vi "Memory.Pointer.Allocate.vi"(7 "allocation limit (2^31: 2GiB)":u64=2147483647 format="%08x bytes", 8 "error in (no error)":errorcluster, 10 "size":u64 format="%d bytes", 11 "Pointer in":refnum<class "Memory.Pointer.Void.lvclass">) -> (0 "error out":errorcluster, 2 "allocated size":u64 format="%0d bytes", 3 "Pointer out":refnum<class "Memory.Pointer.Void.lvclass">)   [LabVIEW 2016, in "LabVIEW Memory Manager.lvlib" / "Memory.Pointer.Void.lvclass"]
uses:
  Memory.Pointer.Void.lvclass
  Memory.Pointer.Void.lvclass/Memory.Pointer.Void.ctl
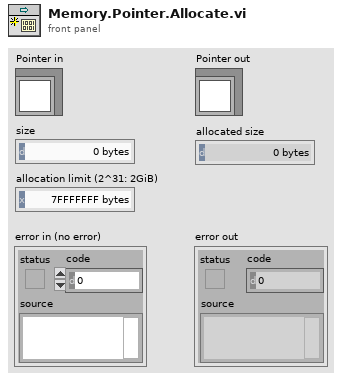
[diagram p1: front panel]
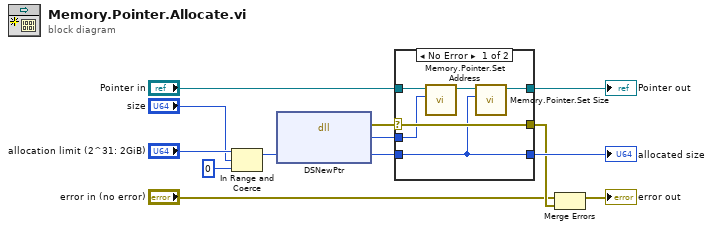
[diagram p0: block diagram]
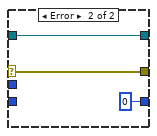
[diagram p2: hidden frame]
diagram:
  n1 = In Range and Coerce(upper limit="allocation limit (2^31: 2GiB)", x="size", lower limit=u64 0) -> (coerced(x)=w5:u64)  [unwired: 1 out]
  n2 = dll-call lib="LabVIEW" fn="DSNewPtr"("size"=w5) -> (error out=w7:errorcluster, "pointer"=w9:u64, "size"=w8:u64)  [unwired: 3 in, 1 out]
  n3 = case shown="No Error" w7 {
    selector: w7 -> [w16 w22]
    tunnel: "Pointer in" -> [w19 w21]
    tunnel: w9 -> [w14 _]
    tunnel: [w17 w21] -> w12
    tunnel: w8 -> [w15 _]
    tunnel: [w16 w22] -> w4
    tunnel: [w15 i64 0 ("size")] -> w13
    frame No Error {
      n4 = call "Memory.Pointer.Set Address.vi"("address"=w14, "Pointer in"=w19) -> ("Pointer out"=w18:refnum<class "Memory.Pointer.Void.lvclass">)  [unwired: 8 in, 1 out]
      n5 = call "Memory.Pointer.Set Size.vi"("size"=w15, "Pointer in"=w18) -> ("Pointer out"=w17:refnum<class "Memory.Pointer.Void.lvclass">)  [unwired: 8 in, 1 out]
    }
    frame Error {
    }
  }
  "Pointer out" <- w12
  "allocated size" <- w13
  n6 = Merge Errors("error in (no error)", w4) -> (→"error out":errorcluster)
